vi "Max Block Count (Transfer).vi"(8 "error in (no error)":errorcluster, 10 "largest block count in (0)":u64, 11 "Transfer in":T1 {"channel blocks"."string descriptor"."buffer offset" format="%d bytes"; "channel blocks"."engine descriptor"."buffer offset" format="%d bytes"}) -> (0 "error out":errorcluster, 2 "largest block count out":u64, 3 "Transfer out":T1 {"channel blocks"."string descriptor"."buffer offset" format="%d bytes"; "channel blocks"."engine descriptor"."buffer offset" format="%d bytes"})   [LabVIEW 2017, in "DSF Core.lvlib"]
uses:
  DSF Core.lvlib
  Controls/DSF Engine Transfer Configuration.ctl
  Controls/DSF Byte Order.ctl
  Controls/DSF Engine Channel Configuration.ctl
  Controls/DSF Channel Buffer Descriptor.ctl
  Controls/DSF Data Type.ctl
  Controls/DSF Settings Info.ctl
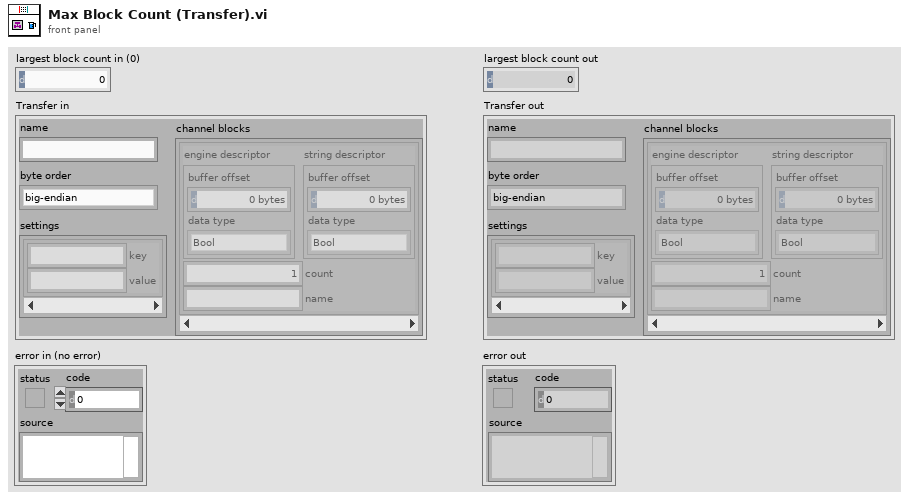
[diagram p1: front panel]
types:
  T1 = typedef "DSF Core.lvlib/DSF Engine Transfer Configuration.ctl" = cluster{"name":string, "byte order":T2, "channel blocks":T3[], "settings":T6}
  T2 = typedef "DSF Core.lvlib/DSF Byte Order.ctl" = enum8{"big-endian", "little-endian"}
  T3 = typedef "DSF Core.lvlib/DSF Engine Channel Configuration.ctl" = cluster{"engine descriptor":T4, "string descriptor":T4, "count":u64, "name":string}
  T4 = typedef "DSF Core.lvlib/DSF Channel Buffer Descriptor.ctl" = cluster{"buffer offset":u64, "data type":T5}
  T5 = typedef "DSF Core.lvlib/DSF Data Type.ctl" = enum8{"Bool", "SGL", "DBL", "I8", "I16", "I32", "I64", "U8", "U16", "U32", "U64"}
  T6 = typedef "DSF Core.lvlib/DSF Settings Info.ctl" = cluster{"key":string, "value":string}[]
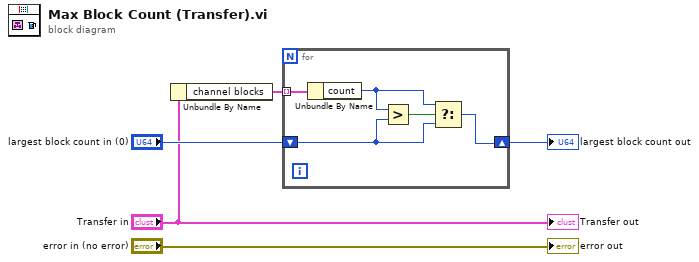
[diagram p0: block diagram]
diagram:
  n1 = Unbundle By Name("Transfer in") -> ("channel blocks"=w1:T3[])
  n2 = for {
    tunnel: w1 -> [w10] mode=indexing
    shift-right: [w6] -> w3
    shift-left: "largest block count in (0)" -> [w7]
    n3 = Unbundle By Name(w10) -> ("count"=w8:u64)
    n4 = Greater?(x=w8, y=w7) -> (0:w9:bool)
    n5 = Select(t=w8, s=w9, f=w7) -> (s? t:f=w6:u64)
  }
  "largest block count out" <- w3
  "error out" <- "error in (no error)"
  "Transfer out" <- "Transfer in"
